vi "SV TDMS Read DBL Array (1 Ch).vi"(0 "tdms file":refnum<k34>, 1 "offset (0)":i64, 2 "count (-1: all)":i64=-1, 5 "group name in":string, 7 "channel name in":string, 11 "error in":errorcluster) -> (3 "scale labels":T1, 4 "tdms file out":refnum<k34>, 6 "group name out":string, 8 "channel name out":string, 10 "scaled signal [EU]":dbl[](array[numeric]), 13 "channel description":string, 14 "eof":bool, 15 "error out":errorcluster)   [LabVIEW 2017]
uses:
  <vilib>/addons/_NISVFA/_Shared subVIs/Controls/NI Channel Properties.ctl
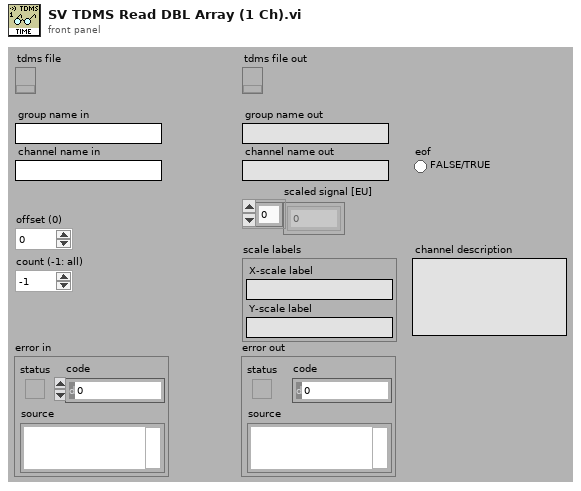
[diagram p1: front panel]
types:
  T1 = cluster{"X-scale label":string, "Y-scale label":string}
  T2 = typedef "NI Channel Properties.ctl" = u16
  T3 = cluster{"scale label with units":string, "scale label with units":string}
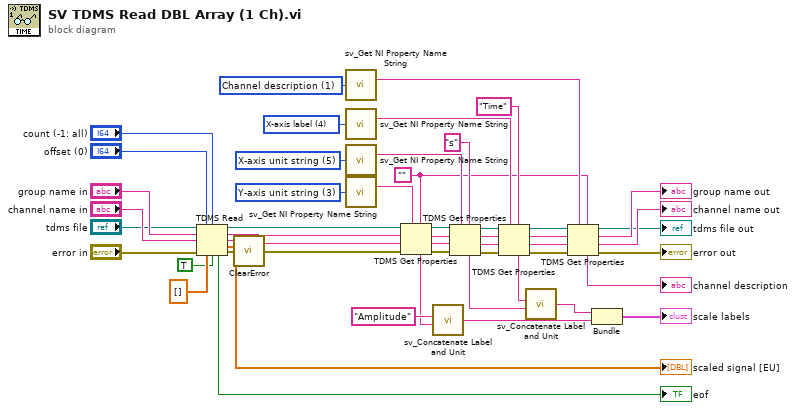
[diagram p0: block diagram]
diagram:
  w10 = T2 1 items=["Channel name", "Channel description", "Y-axis label", "Y-axis unit string", "X-axis label", "X-axis unit string", "x0", "dx", "Number of samples", "X channel", "Filter settled", "dB reference", "Window", "Window parameter", "Window size", "FFT size", "Peak units", "Spectrum type", "Magnitude scale", "Spectral density", "Sensor sensitivity (mV/EU)", "X-axis domain", "LabVIEW datatype"] ("property")
  w8 = "" ("data type")
  w32 = T2 3 items=["Channel name", "Channel description", "Y-axis label", "Y-axis unit string", "X-axis label", "X-axis unit string", "x0", "dx", "Number of samples", "X channel", "Filter settled", "dB reference", "Window", "Window parameter", "Window size", "FFT size", "Peak units", "Spectrum type", "Magnitude scale", "Spectral density", "Sensor sensitivity (mV/EU)", "X-axis domain", "LabVIEW datatype"] ("property")
  w33 = T2 4 items=["Channel name", "Channel description", "Y-axis label", "Y-axis unit string", "X-axis label", "X-axis unit string", "x0", "dx", "Number of samples", "X channel", "Filter settled", "dB reference", "Window", "Window parameter", "Window size", "FFT size", "Peak units", "Spectrum type", "Magnitude scale", "Spectral density", "Sensor sensitivity (mV/EU)", "X-axis domain", "LabVIEW datatype"] ("property")
  w34 = T2 5 items=["Channel name", "Channel description", "Y-axis label", "Y-axis unit string", "X-axis label", "X-axis unit string", "x0", "dx", "Number of samples", "X channel", "Filter settled", "dB reference", "Window", "Window parameter", "Window size", "FFT size", "Peak units", "Spectrum type", "Magnitude scale", "Spectral density", "Sensor sensitivity (mV/EU)", "X-axis domain", "LabVIEW datatype"] ("property")
  n1 = TDMS Read(0:"tdms file", 1:"offset (0)", 2:"count (-1: all)", 5:"group name in", 7:"channel name in", 11:"error in", 12:dbl[] [] ("scaled signal [EU]"), 13:TRUE ("return channels in file order? (F)")) -> (4:w25:refnum<k34>, 6:w26:string, 8:w24:string, 10:→"scaled signal [EU]":dbl[], 14:→"eof":bool, 15:w2:errorcluster)
  n2 = call <vilib>:"ClearError.vi"("error in (no error)"=w2) -> ("error out"=w27:errorcluster)
  n3 = call <vilib>:"sv_Get NI Property Name String.vi"("property"=w10) -> ("TDMS property name"=w9:string)  [unwired: 13 in, 1 out]
  n4 = call <vilib>:"sv_Get NI Property Name String.vi"("property"=w33) -> ("TDMS property name"=w31:string)  [unwired: 13 in, 1 out]
  n5 = call <vilib>:"sv_Get NI Property Name String.vi"("property"=w34) -> ("TDMS property name"=w30:string)  [unwired: 13 in, 1 out]
  n6 = call <vilib>:"sv_Get NI Property Name String.vi"("property"=w32) -> ("TDMS property name"=w15:string)  [unwired: 13 in, 1 out]
  n7 = TDMS Get Properties(5:w8, 7:w15, 8:w27, 9:w24, 10:w26, 11:w25) -> (0:w23:errorcluster, 1:w16:string, 2:w17:string, 3:w18:refnum<k34>, 4:w3:string)  [unwired: 1 out]
  n8 = call <vilib>:"sv_Concatenate Label and Unit.vi"("unit string"=w3, "label"="Amplitude") -> ("scale label with units"=w6:string)  [unwired: 4 in]
  n9 = TDMS Get Properties(5:"s" ("channel name"), 7:w30, 8:w23, 9:w16, 10:w17, 11:w18) -> (0:w39:errorcluster, 1:w40:string, 2:w41:string, 3:w42:refnum<k34>, 4:w28:string)  [unwired: 1 out]
  n10 = TDMS Get Properties(5:"Time" ("group name"), 7:w31, 8:w39, 9:w40, 10:w41, 11:w42) -> (0:w19:errorcluster, 1:w20:string, 2:w21:string, 3:w22:refnum<k34>, 4:w29:string)  [unwired: 1 out]
  n11 = call <vilib>:"sv_Concatenate Label and Unit.vi"("unit string"=w28, "label"=w29) -> ("scale label with units"=w4:string)  [unwired: 4 in]
  n12 = TDMS Get Properties(5:w8, 7:w9, 8:w19, 9:w20, 10:w21, 11:w22) -> (0:→"error out":errorcluster, 1:→"channel name out":string, 2:→"group name out":string, 3:→"tdms file out":refnum<k34>, 4:→"channel description":string)  [unwired: 1 out]
  n13 = Bundle("scale label with units"=w4, "scale label with units"=w6) -> (→"scale labels":T3)  [unwired: 1 in]
